vi "Measurement Logic.vi"(8 "error in":errorcluster, 10 "Measurement Context":refnum<class "MeasurementContext.lvclass">, 11 "Measurement Configuration":T3={"Number of channels to measure"=0, "Full scale range"=10.0, "Analog source input channels"=[], "Analog source resource names"=[], "Frequency"=1000.0, "Amplitude"=-1.0, "Digital capture resource name"="", "Digital capture sample rate"=800000.0, "Digital capture samples"=800000}) -> (0 "error out":errorcluster, 2 "Measurement Context out":refnum<class "MeasurementContext.lvclass">, 3 "Measurement Results":T2)   [LabVIEW 2021, in "adc_acMultiChannelMeasurement.lvlib"]
uses:
  adc_acMultiChannelMeasurement.lvlib
  Measurement Configuration.ctl
  Measurement Results.ctl
  <vilib>/MeasurementLink/MeasurementLink Measurement Server/Classes/MeasurementContext/MeasurementContext.lvclass
  shared/controls/HW Sync Commands.ctl
  <instrlib>/niDigital/niDigital.llb/niDigital Trigger Digital Edge - Edge.ctl
  <vilib>/DAQmx/create/channels.llb/DAQmx Create Channel (AO-Voltage-Basic).vi
  <vilib>/DAQmx/configure/timing.llb/DAQmx Timing (Sample Clock).vi
  <vilib>/DAQmx/create/channels.llb/DAQmx Create Channel (AO-FuncGen).vi
  <vilib>/FPGAPlugInAG/Dynamic/niLvFpga_Close_Dynamic.vi
  <vilib>/rvi/interface/nirviCloseFPGA/nirviCloseFPGA.xnode
  <resource>/objmgr/daqmx.rc
panel:
  in  "Pin config":T1(array[cluster])=[{"Pin"="RESET", "Current Limit"=0.01, "Voltage Level"=3.3}, {"Pin"="SCLK", "Current Limit"=0.01, "Voltage Level"=3.3}, {"Pin"="CS", "Current Limit"=0.01, "Voltage Level"=3.3}, {"Pin"="WR", "Current Limit"=0.01, "Voltage Level"=3.3}, {"Pin"="CONVST", "Current Limit"=0.01, "Voltage Level"=0.0}, {"Pin"="REFSEL", "Current Limit"=0.01, "Voltage Level"=3.3}, {"Pin"="STBY", "Current Limit"=0.01, "Voltage Level"=3.3}, {"Pin"="SERPAR", "Current Limit"=0.01, "Voltage Level"=0.0}, {"Pin"="RANGE", "Current Limit"=0.01, "Voltage Level"=0.0}, {"Pin"="OS0", "Current Limit"=0.01, "Voltage Level"=0.0}, {"Pin"="OS1", "Current Limit"=0.01, "Voltage Level"=0.0}, {"Pin"="OS2", "Current Limit"=0.01, "Voltage Level"=0.0}, {"Pin"="RESET", "Current Limit"=0.01, "Voltage Level"=0.0}]
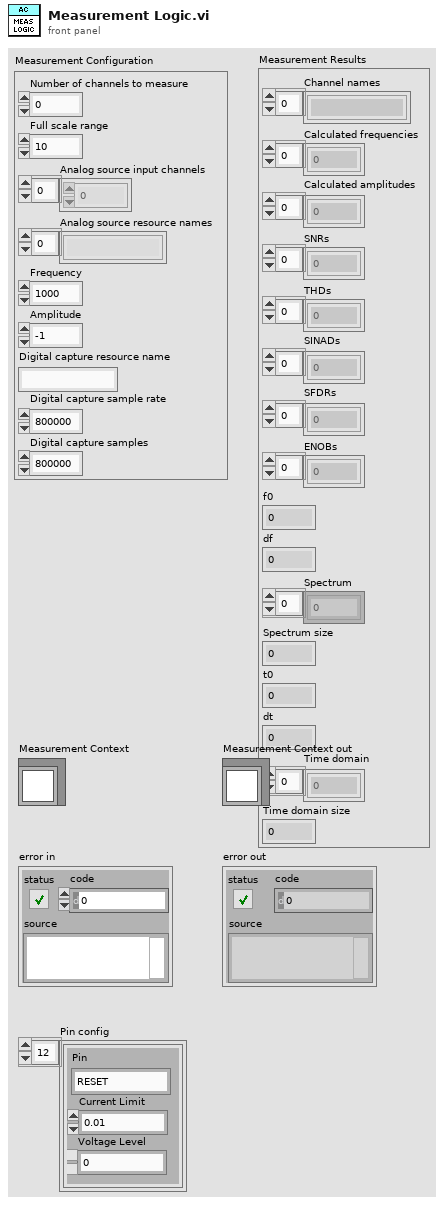
[diagram p1: front panel]
types:
  T1 = cluster{"Pin":string, "Current Limit":dbl, "Voltage Level":dbl}[]
  T2 = typedef "adc_acMultiChannelMeasurement.lvlib/Measurement Results.ctl" = cluster{"Channel names":string[], "Calculated frequencies":dbl[], "Calculated amplitudes":dbl[], "SNRs":dbl[], "THDs":dbl[], "SINADs":dbl[], "SFDRs":dbl[], "ENOBs":dbl[], "f0":dbl, "df":dbl, "Spectrum":dbl[], "Spectrum size":i32, "t0":dbl, "dt":dbl, "Time domain":dbl[], "Time domain size":i32}
  T3 = typedef "adc_acMultiChannelMeasurement.lvlib/Measurement Configuration.ctl" = cluster{"Number of channels to measure":i32, "Full scale range":dbl, "Analog source input channels":i32[], "Analog source resource names":string[], "Frequency":dbl, "Amplitude":dbl, "Digital capture resource name":string, "Digital capture sample rate":dbl, "Digital capture samples":u32}
  T4 = typedef "HW Sync Commands.ctl" = enum16{"NoAction", "GenerationStarted", "AcquisitionCompleted", "GenerationErrored"}
  T5 = cluster{"DSG Session":refnum<k21>, "DPI Bitfile reference":refnum<k20>, "DPI Session":refnum<k15>}
  T6 = typedef "niDigital Trigger Digital Edge - Edge.ctl" = i32
  T7 = typedef "Sync Commands.ctl" = enum16{"NoAction", "GenerationStarted", "AcquisitionCompleted", "GenerationErrored"}
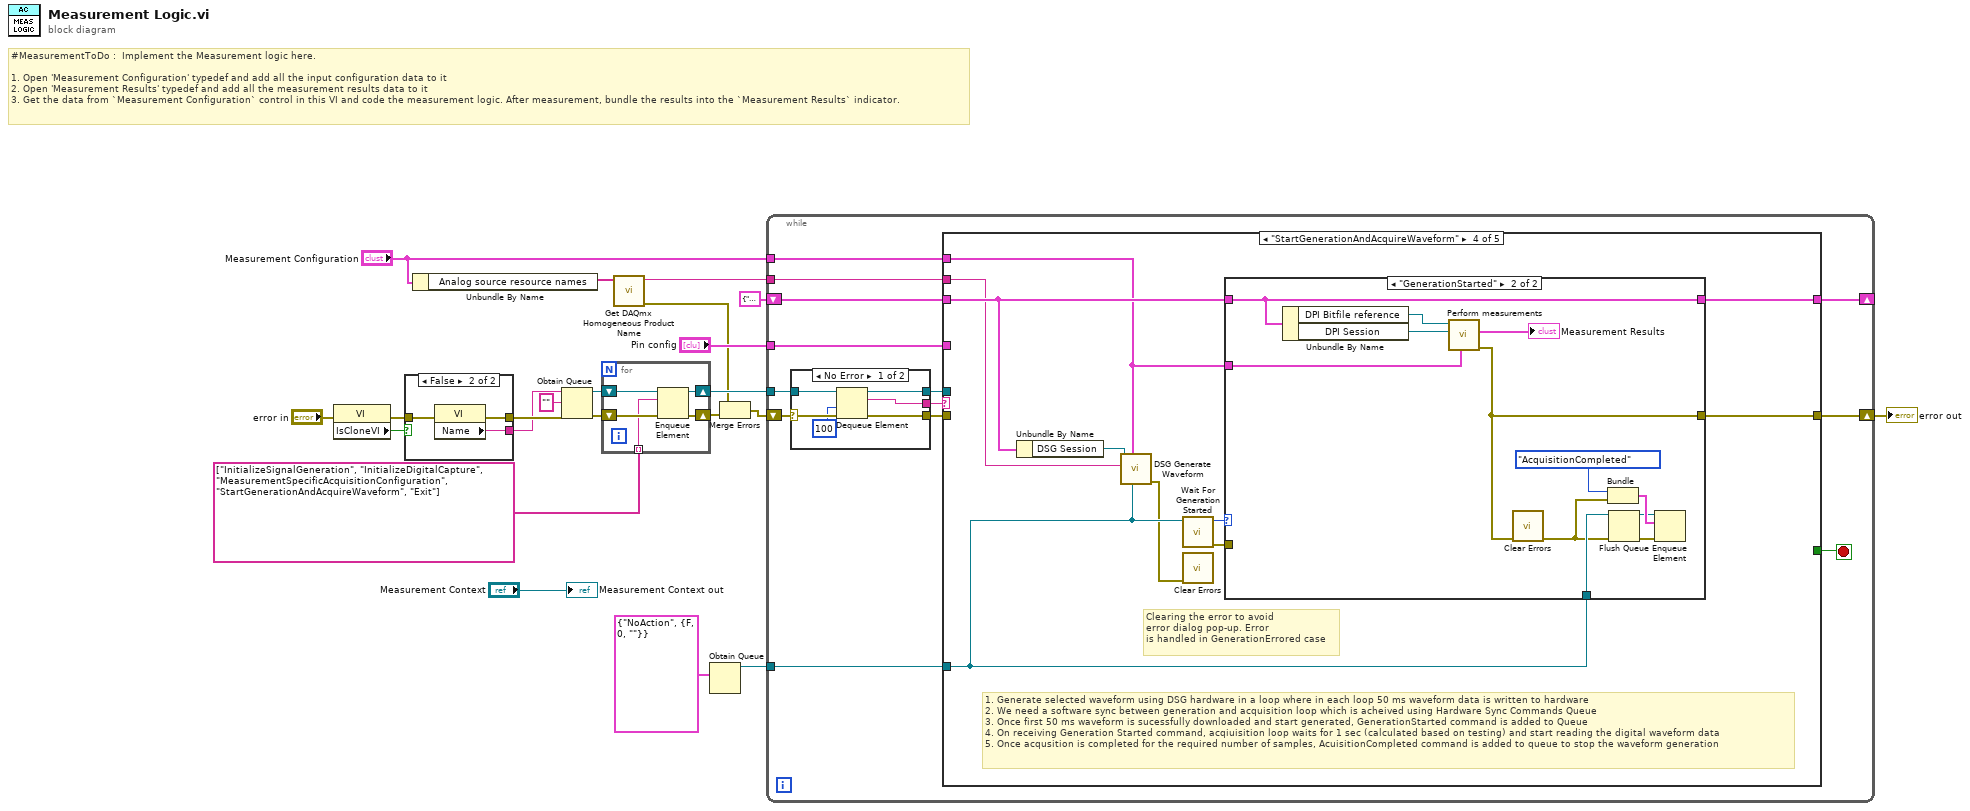
[diagram p0: block diagram]
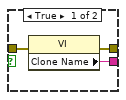
[diagram p2: hidden frame]
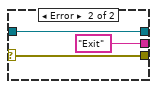
[diagram p3: hidden frame]
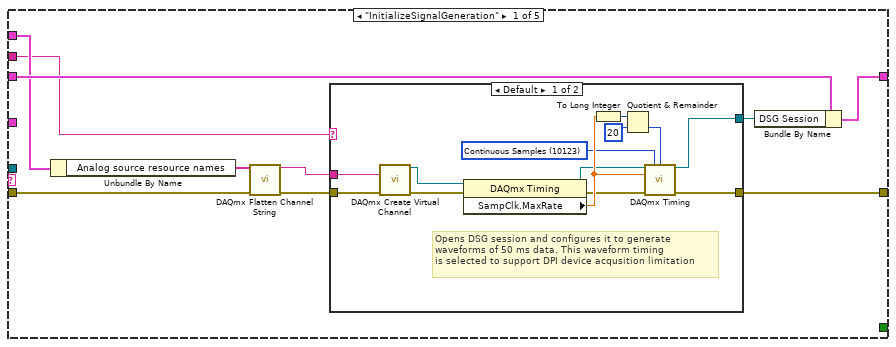
[diagram p4: hidden frame]
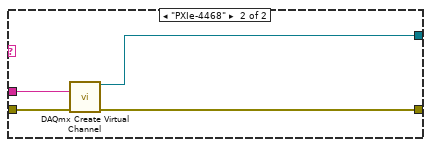
[diagram p5: hidden frame]
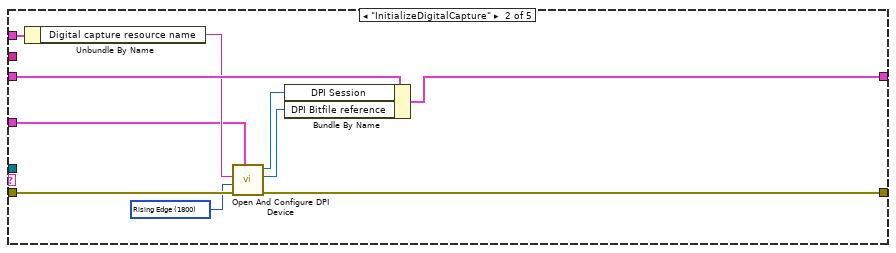
[diagram p6: hidden frame]
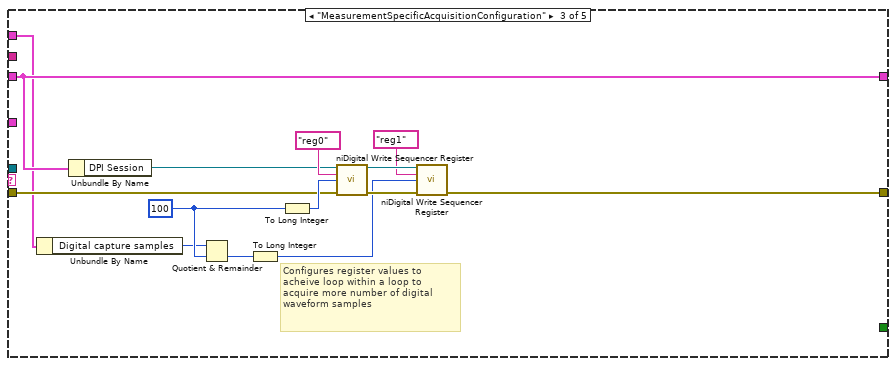
[diagram p7: hidden frame]
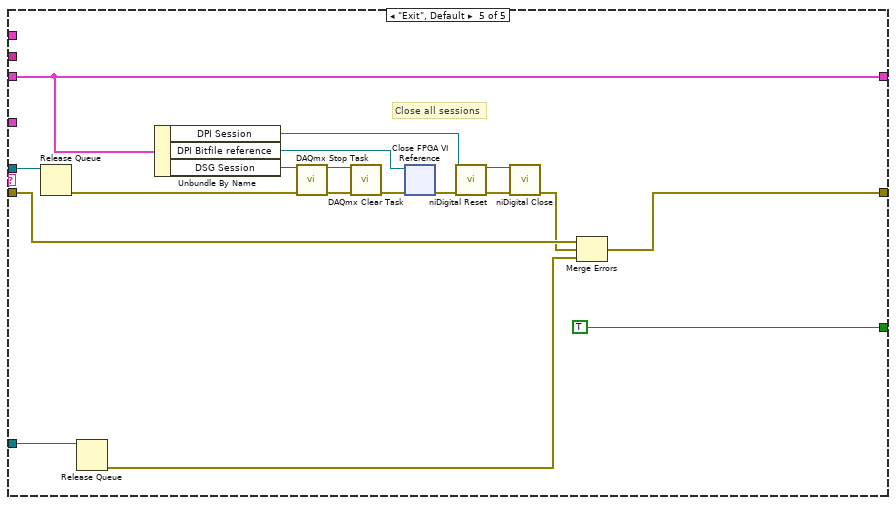
[diagram p9: hidden frame]
diagram:
  # "#MeasurementToDo :  Implement the Measurement logic here.\n\n1. Open 'Measurement Configuration' typedef and add all the input configuration data to it\n2. Open 'Measurement Results' typedef and add all the measurement results data to it\n3. Get the data from `Measurement Configuration` control in this VI and code the measurement logic. After measurement, bundle the results into the `Measurement Results` indicator."
  n1 = property class="VI"(error in="error in") -> (error out=w11:errorcluster, "IsCloneVI"=w12:bool)  [unwired: 1 in, 1 out]
  n2 = case shown="False" w12 {
    tunnel: [w25 w28] -> w9
    tunnel: [w24 w27] -> w8
    tunnel: w11 -> [w23 w26]
    frame True {
      n3 = property class="VI"(error in=w23) -> (error out=w25:errorcluster, "Clone Name"=w24:string)  [unwired: 1 in, 1 out]
    }
    frame False {
      n4 = property class="VI"(error in=w26) -> (error out=w28:errorcluster, "Name"=w27:string)  [unwired: 1 in, 1 out]
    }
  }
  n5 = Unbundle By Name("Measurement Configuration") -> ("Analog source resource names"=w5:string[])
  n6 = Obtain Queue(name (unnamed)=w8, element data type="", error in (no error)=w9) -> (queue out=w20:refnum<queue>, error out=w7:errorcluster)  [unwired: 2 in, 1 out]
  n7 = for {
    shift-right: [w31] -> w19
    shift-left: w20 -> [w33]
    shift-right: [w30] -> w2
    shift-left: w7 -> [w32]
    tunnel: string[] ["InitializeSignalGeneration", "InitializeDigitalCapture", "MeasurementSpecificAcquisitionConfiguration", "StartGenerationAndAcquireWaveform", "Exit"] ("Step sequence") -> [w29] mode=indexing
    n8 = Enqueue Element(queue=w33, element=w29, error in (no error)=w32) -> (queue out=w31:refnum<queue>, error out=w30:errorcluster)  [unwired: 1 in, 1 out]
  }
  n9 = call "Get DAQmx Homogeneous Product Name.vi"("Analog source resource names"=w5) -> ("error out"=w3:errorcluster, "Device model"=w4:string)  [unwired: 9 in]
  n10 = Obtain Queue(element data type=cluster{"Status":T4, "Error":errorcluster} {"Status"=enum."NoAction", "Error"={"status"=FALSE, "code"=0, "source"=""}}) -> (queue out=w15:refnum<queue>)  [unwired: 4 in, 2 out]
  n11 = Merge Errors(w3, w2) -> (w1:errorcluster)
  n12 = while {
    tunnel: w19 -> [w38]
    shift-right: [w46] -> w13
    shift-left: w1 -> [w39]
    tunnel: "Measurement Configuration" -> [w44]
    shift-right: [w42] -> _
    shift-left: T5 {"DSG Session"="", "DPI Bitfile reference"=refnum, "DPI Session"=""} ("output cluster") -> [w43]
    tunnel: "Pin config" -> [w41]
    tunnel: w15 -> [w40]
    tunnel: w4 -> [w34]
    stop <- w45 stop-if-true
    n13 = case shown="No Error" w39 {
      selector: w39 -> [w50 w54]
      tunnel: w38 -> [w52 w53]
      tunnel: [w51 "Exit" ("t")] -> w37
      tunnel: [w49 w54] -> w36
      tunnel: [w47 w53] -> w35
      frame No Error {
        n14 = Dequeue Element(queue=w52, timeout in ms (-1)=100, error in (no error)=w50) -> (queue out=w47:refnum<queue>, element=w51:string, error out=w49:errorcluster)  [unwired: 1 out]
      }
      frame Error {
      }
    }
    n15 = case shown="\"StartGenerationAndAcquireWaveform\"" w37 {
      tunnel: [w65 w88 w96 w116 w132] -> w46
      tunnel: w36 -> [w56 w87 w97 _ w134]
      tunnel: [_ _ _ _ TRUE] -> w45
      tunnel: w44 -> [w62 w92 w95 w109 _]
      tunnel: w43 -> [w64 w90 w101 w115 w142]
      tunnel: [w63 w91 w101 w114 w142] -> w42
      tunnel: w41 -> [_ w83 _ _ _]
      tunnel: w40 -> [_ _ _ w113 w137]
      tunnel: w35 -> [_ _ _ _ w136]
      tunnel: w34 -> [w60 _ _ w108 _]
      frame "InitializeSignalGeneration" {
        n16 = Unbundle By Name(w62) -> ("Analog source resource names"=w59:string[])
        n17 = call <vilib>:"DAQmx Flatten Channel String.vi"("names in"=w59, "error in"=w56) -> ("names out"=w58:string, "error out"=w57:errorcluster)  [unwired: 12 in]
        n18 = case shown="Default" w60 {
          tunnel: w58 -> [w78 w79]
          tunnel: w57 -> [w77 w82]
          tunnel: [w76 w81] -> w65
          tunnel: [w66 w80] -> w61
          frame Default {
            w67 = 10123 items=["Finite Samples"=10178, "Continuous Samples"=10123, "Hardware Timed Single Point"=12522] ("sample mode")
            # "Opens DSG session and configures it to generate\nwaveforms of 50 ms data. This waveform timing\nis selected to support DPI device acqusition limitation"
            n19 = call-poly <vilib>:"DAQmx Create Virtual Channel.vi"("physical channels"=w78, "error in"=w77) -> ("task out"=w75:refnum<k21>, "error out"=w74:errorcluster)  [unwired: 12 in]
            n20 = property class="DAQmx Timing"(reference=w75, error in=w74) -> (reference out=w70:refnum<k21>, error out=w71:errorcluster, "SampClk.MaxRate"=w72:dbl)
            n21 = To Long Integer(number=w72) -> (32bit integer=w68:i32)
            n22 = Quotient & Remainder(x=w68, y=20) -> (floor(x/y)=w73:i32)  [unwired: 1 out]
            n23 = call-poly <vilib>:"DAQmx Timing.vi"("task/channels in"=w70, "sample mode"=w67, "samples per channel"=w73, "rate"=w72, "error in"=w71) -> ("task out"=w66:refnum<k21>, "error out"=w76:errorcluster)  [unwired: 9 in]
          }
          frame "PXIe-4468" {
            n24 = call-poly <vilib>:"DAQmx Create Virtual Channel.vi"("physical channels"=w79, "error in"=w82) -> ("task out"=w80:refnum<k21>, "error out"=w81:errorcluster)  [unwired: 12 in]
          }
        }
        n25 = Bundle By Name(cluster=w64, "DSG Session"=w61) -> (w63:T5)
      }
      frame "InitializeDigitalCapture" {
        w84 = T6 1800 items=["Rising Edge"=1800, "Falling Edge"=1801] ("TriggerEdge")
        n26 = Unbundle By Name(w92) -> ("Digital capture resource name"=w86:string)
        n27 = call "Open And Configure DPI Device.vi"("Pin config"=w83, "error in (no error)"=w87, "TriggerEdge"=w84, "DPI resource name"=w86) -> ("error out"=w88:errorcluster, "DPI Bitfile reference"=w89:refnum<k20>, "DPI Session"=w85:refnum<k15>)  [unwired: 5 in]
        n28 = Bundle By Name(cluster=w90, "DPI Session"=w85, "DPI Bitfile reference"=w89) -> (w91:T5)
      }
      frame "MeasurementSpecificAcquisitionConfiguration" {
        w100 = u32 100 ("value")
        # "Configures register values to acheive loop within a loop to acquire more number of digital waveform samples"
        n29 = Unbundle By Name(w95) -> ("Digital capture samples"=w94:u32)
        n30 = Unbundle By Name(w101) -> ("DPI Session"=w98:refnum<k15>)
        n31 = Quotient & Remainder(x=w94, y=w100) -> (floor(x/y)=w93:u32)  [unwired: 1 out]
        n32 = To Long Integer(number=w93) -> (32bit integer=w99:i32)
        n33 = To Long Integer(number=w100) -> (32bit integer=w102:i32)
        n34 = call <instrlib>:"niDigital Write Sequencer Register.vi"("instrument handle"=w98, "sequencer register"="reg0", "value"=w102, "error in"=w97) -> ("instrument handle out"=w106:refnum<k15>, "error out"=w105:errorcluster)  [unwired: 10 in]
        n35 = call <instrlib>:"niDigital Write Sequencer Register.vi"("instrument handle"=w106, "sequencer register"="reg1", "value"=w99, "error in"=w105) -> ("error out"=w96:errorcluster)  [unwired: 10 in, 1 out]
      }
      frame "StartGenerationAndAcquireWaveform" {
        # "1. Generate selected waveform using DSG hardware in a loop where in each loop 50 ms waveform data is written to hardware\n2. We need a software sync between generation and acquisition loop which is acheived using Hardware Sync Commands Queue\n3. Once first 50 ms waveform is sucessfully downloaded and start generated, GenerationStarted command is added to Queue\n4. On receiving Generation Started command, acqiuisition loop waits for 1 sec (calculated based on testing) and start reading the digital waveform data\n5. Once acqusition is completed for the required number of samples, AcuisitionCompleted command is added to queue to stop the waveform generation"
        # "Clearing the error to avoid\nerror dialog pop-up. Error\nis handled in GenerationErrored case"
        n36 = Unbundle By Name(w115) -> ("DSG Session"=w107:refnum<k21>)
        n37 = call "DSG Generate Waveform.vi"("hardware commands sync queue"=w113, "measurement configuration"=w109, "DAQmx product name"=w108, "DSG task in"=w107) -> ("error out"=w110:errorcluster)  [unwired: 6 in, 1 out]
        n38 = call "Wait For Generation Started.vi"("hardware commands sync queue"=w113) -> ("error out"=w111:errorcluster, "Status"=w112:T7)  [unwired: 9 in]
        n39 = call <vilib>:"Clear Errors.vi"("error in (no error)"=w110) -> ()  [unwired: 5 in, 2 out]
        n40 = case shown="\"GenerationStarted\"" w112 {
          tunnel: [w117 w119] -> w116
          tunnel: w113 -> [_ w126]
          tunnel: w115 -> [w118 w128]
          tunnel: [w118 w128] -> w114
          tunnel: w109 -> [_ w121]
          tunnel: w111 -> [w117 _]
          frame Default {
          }
          frame "GenerationStarted" {
            n41 = Unbundle By Name(w128) -> ("DPI Bitfile reference"=w123:refnum<k20>, "DPI Session"=w122:refnum<k15>)
            n42 = call "Perform measurements.vi"("Measurement configuration"=w121, "DPI Session"=w122, "DPI Bitfile reference"=w123) -> ("error out"=w119:errorcluster, "Measurement results"=→"Measurement Results":T2)  [unwired: 7 in]
            n43 = call <vilib>:"Clear Errors.vi"("error in (no error)"=w119) -> ("error out"=w125:errorcluster)  [unwired: 5 in, 1 out]
            n44 = Bundle("element"=HW_Sync_Commands."AcquisitionCompleted", "error out"=w125) -> (w129:cluster{"element":T4, "error out":errorcluster})  [unwired: 1 in]
            n45 = Flush Queue(queue=w126, error in (no error)=w125) -> (queue out=w127:refnum<queue>, error out=w124:errorcluster)  [unwired: 1 out]
            n46 = Enqueue Element(queue=w127, element=w129, error in (no error)=w124) -> ()  [unwired: 1 in, 3 out]
          }
        }
      }
      frame "Exit", Default {
        # "Close all sessions"
        n47 = Release Queue(queue=w136) -> (error out=w135:errorcluster)  [unwired: 2 in, 2 out]
        n48 = Release Queue(queue=w137) -> (error out=w131:errorcluster)  [unwired: 2 in, 2 out]
        n49 = Unbundle By Name(w142) -> ("DPI Session"=w141:refnum<k15>, "DPI Bitfile reference"=w143:refnum<k20>, "DSG Session"=w147:refnum<k21>)
        n50 = call <vilib>:"DAQmx Stop Task.vi"("task/channels in"=w147, "error in"=w135) -> ("task out"=w146:refnum<k21>, "error out"=w145:errorcluster)  [unwired: 12 in]
        n51 = call <vilib>:"DAQmx Clear Task.vi"("task in"=w146, "error in"=w145) -> ("error out"=w144:errorcluster)  [unwired: 13 in]
        n52 = xnode "Close FPGA VI Reference"("FPGA VI Reference In"=w143, "error in"=w144) -> ("error out"=w138:errorcluster)
        n53 = call <instrlib>:"niDigital Reset.vi"("instrument handle in"=w141, "error in"=w138) -> ("instrument handle out"=w139:refnum<k15>, "error out"=w140:errorcluster)  [unwired: 12 in]
        n54 = call <instrlib>:"niDigital Close.vi"("instrument handle"=w139, "error in"=w140) -> ("error out"=w133:errorcluster)  [unwired: 13 in]
        n55 = Merge Errors(w134, w133, w131) -> (w132:errorcluster)
      }
    }
  }
  "error out" <- w13
  "Measurement Context out" <- "Measurement Context"
